vi "XControl Resize.vi"(8 "Progress Bar Refnum":refnum<vi>, 9 "Glyph Refnum":refnum<vi>, 10 "State":T1={"Window Handle"=refnum, "Maximum"=100, "State Change Action"=enum."No Action", "Running"=FALSE, "Visable Items"={"Label"=TRUE, "Caption"=FALSE}, "Value"=0, "Show Progress Bar"=FALSE}, 11 "Container State":T3) -> ()   [LabVIEW 2011, in "Taskbar Progress Bar.xctl"]
uses:
  Taskbar Progress Bar.xctl
  <vilib>/_xctls/Container State.ctl
  Abilities/PB State.ctl
  TypeDefs/Dispaly State Change Methods.ctl
  <vilib>/Utility/miscctls.llb/LVBoundsTypeDef.ctl
  <vilib>/_xctls/XControlSupport.lvlib
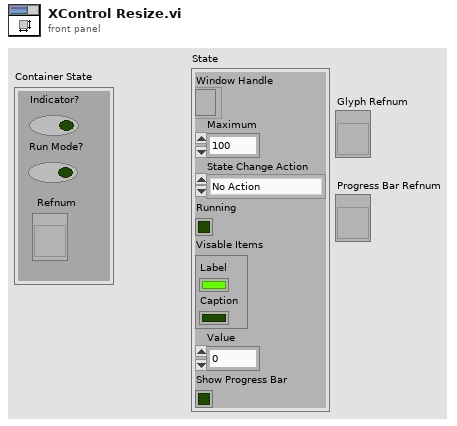
[diagram p1: front panel]
types:
  T1 = typedef "Taskbar Progress Bar.xctl/PB State.ctl" = cluster{"Window Handle":refnum<k24>, "Maximum":u64, "State Change Action":T2, "Running":bool, "Visable Items":cluster{"Label":bool, "Caption":bool}, "Value":u64, "Show Progress Bar":bool}
  T2 = typedef "Taskbar Progress Bar.xctl/Dispaly State Change Methods.ctl" = enum16{"No Action", "Created", "Method - Initialize", "Method - Increment", "Method - Pause", "Method - Error", "Method - Finish", "Property - Show Progress Bar"}
  T3 = typedef "XControlSupport.lvlib/Container State.ctl" = cluster{"Indicator?":bool, "Run Mode?":bool, " Refnum":refnum<vi>}
  T4 = typedef "LVBoundsTypeDef.ctl" = cluster{"Width":u32, "Height":u32}
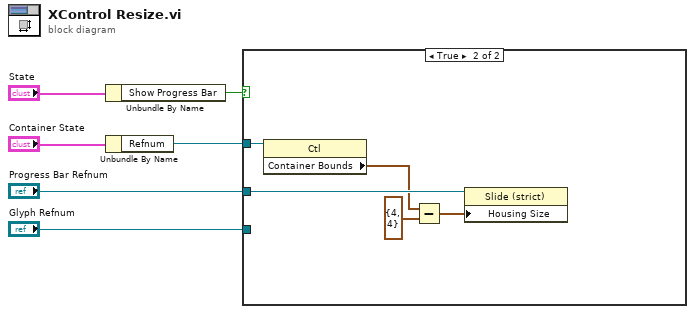
[diagram p0: block diagram]
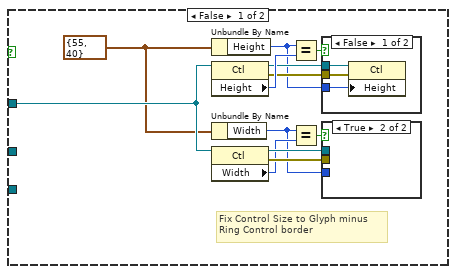
[diagram p2: hidden frame]
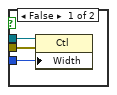
[diagram p3: hidden frame]
diagram:
  n1 = Unbundle By Name("State") -> ("Show Progress Bar"=w3:bool)
  n2 = Unbundle By Name("Container State") -> ("Refnum"=w6:refnum<vi>)
  n3 = case shown="True" w3 {
    tunnel: w6 -> [w18 w28]
    tunnel: "Progress Bar Refnum" -> [_ w29]
    tunnel: "Glyph Refnum" -> [_ _]
    frame False {
      w7 = T4 {"Width"=55, "Height"=40} ("input cluster")
      # "Fix Control Size to Glyph minus \nRing Control border"
      n4 = Unbundle By Name(w7) -> ("Height"=w8:u32)
      n5 = property class="Ctl"(reference=w18) -> (reference out=w10:refnum<vi>, error out=w11:errorcluster, "Height"=w12:u32)  [unwired: 1 in]
      n6 = Unbundle By Name(w7) -> ("Width"=w9:u32)
      n7 = property class="Ctl"(reference=w18) -> (reference out=w17:refnum<vi>, error out=w16:errorcluster, "Width"=w15:u32)  [unwired: 1 in]
      n8 = Equal?(x=w8, y=w12) -> (x = y?=w13:bool)
      n9 = Equal?(x=w9, y=w15) -> (x = y?=w14:bool)
      n10 = case shown="False" w13 {
        tunnel: w10 -> [w24 _]
        tunnel: w11 -> [w23 _]
        tunnel: w8 -> [w22 _]
        frame False {
          n11 = property class="Ctl"(reference=w24, error in=w23, "Height"=w22) -> ()  [unwired: 2 out]
        }
        frame True {
        }
      }
      n12 = case shown="True" w14 {
        tunnel: w17 -> [w21 _]
        tunnel: w16 -> [w20 _]
        tunnel: w9 -> [w19 _]
        frame False {
          n13 = property class="Ctl"(reference=w21, error in=w20, "Width"=w19) -> ()  [unwired: 2 out]
        }
        frame True {
        }
      }
    }
    frame True {
      n14 = property class="Ctl"(reference=w28) -> ("Container Bounds"=w27:T4)  [unwired: 1 in, 2 out]
      n15 = Subtract(x=w27, y=T4 {"Width"=4, "Height"=4}) -> (x-y=w26:T4)
      n16 = property class="Slide (strict)"(reference=w29, "Housing Size"=w26) -> ()  [unwired: 1 in, 2 out]
    }
  }
